vi "Set Switch State.vi"(0 "VISA resource name":refnum<visa-resource-name>, 7 "Switch State":T1, 11 "error in (no error)":errorcluster) -> (4 "VISA resource name out":refnum<visa-resource-name>, 15 "error out":errorcluster)   [LabVIEW 2023, in "ACM Visa Driver.lvlib"]
uses:
  ACM Visa Driver.lvlib
  Controls/ACM Switch States.ctl
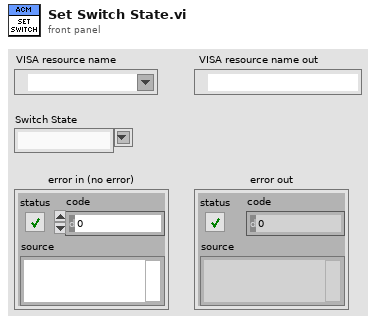
[diagram p1: front panel]
types:
  T1 = typedef "ACM Visa Driver.lvlib/ACM Switch States.ctl" = string
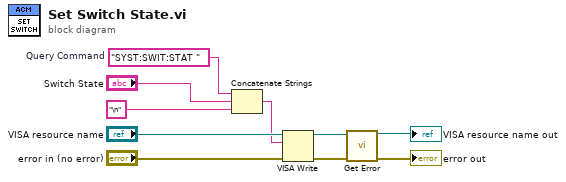
[diagram p0: block diagram]
diagram:
  w7 = "SYST:SWIT:STAT "  # Query Command
  n1 = Concatenate Strings(w7, "Switch State", "\n") -> (w6:string)
  n2 = VISA Write(VISA resource name="VISA resource name", write buffer=w6, error in (no error)="error in (no error)") -> (VISA resource name out=w2:refnum<visa-resource-name>, error out=w9:errorcluster)  [unwired: 1 out]
  n3 = call "Get Error.vi"("VISA resource name"=w2, "error in (no error)"=w9) -> ("VISA resource name out"=→"VISA resource name out":refnum<visa-resource-name>, "error out"=→"error out":errorcluster)  [unwired: 12 in]
